vi "FTW-Container-Equal.vi"(0 "FTW-Container In":variant, 5 "Other Container":variant, 11 "error in":errorcluster) -> (8 "Equal":bool, 15 "error out":errorcluster)   [LabVIEW 2015, in "FTW-Container.lvclass"]
uses:
  FTW-Container.lvclass
  <vilib>/Utility/Data Type/NI_Data Type.lvlib
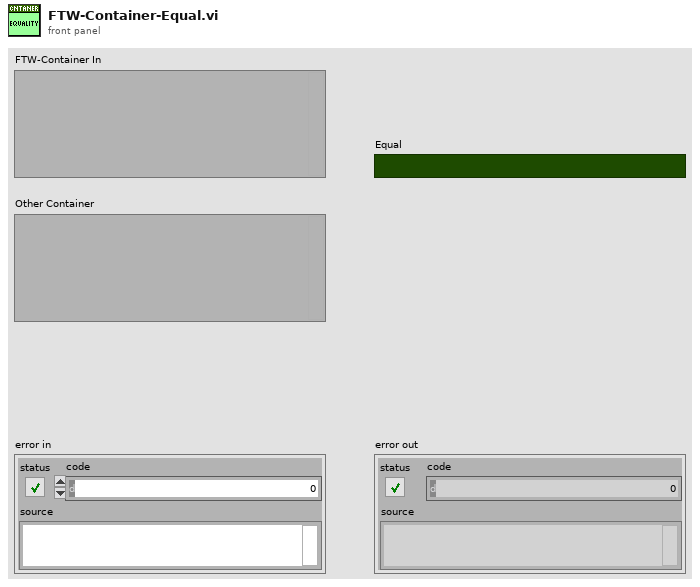
[diagram p1: front panel]
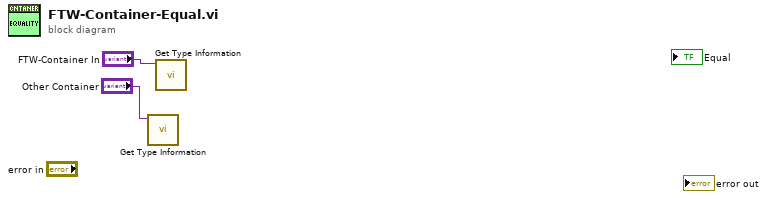
[diagram p0: block diagram]
diagram:
  n1 = call <vilib>:"Get Type Information.vi"("Variant"="Other Container") -> ()  [unwired: 6 in, 5 out]
  n2 = call <vilib>:"Get Type Information.vi"("Variant"="FTW-Container In") -> ()  [unwired: 6 in, 5 out]
